vi "F Dwf Analog Impedance Comp Set.vi"(6 "ohmShortReactance":dbl, 7 "ohmShortResistance":dbl, 8 "error in (no error)":errorcluster, 9 "ohmOpenReactance":dbl, 10 "ohmOpenResistance":dbl, 11 "hdwf":i32) -> (0 "error out":errorcluster, 3 "function return":i32)   [LabVIEW 2021, in "Olasdwf.lvlib"]
doc: "DWFAPI int FDwfAnalogImpedanceCompSet(HDWF hdwf, double ohmOpenResistance, double ohmOpenReactance, double ohmShortResistance, double ohmShortReactance);"
uses:
  Olasdwf.lvlib
  Windows/System32/dwf.dll
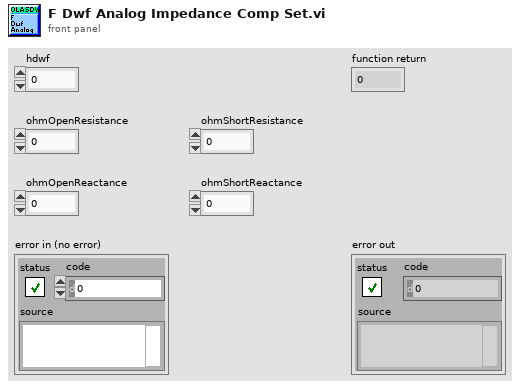
[diagram p1: front panel]
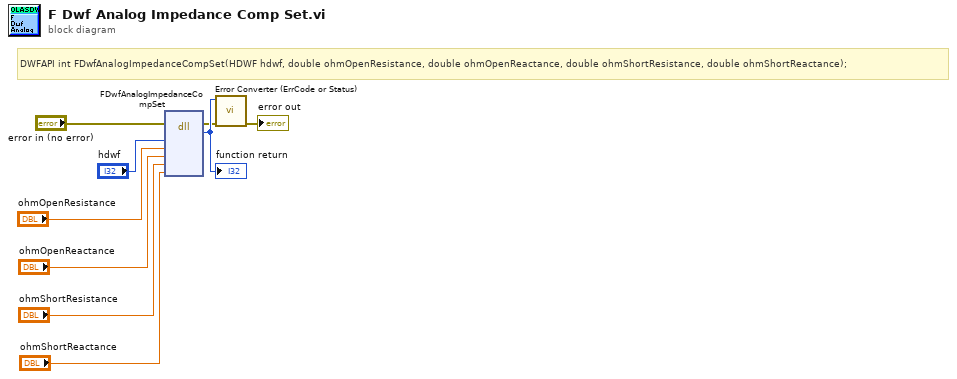
[diagram p0: block diagram]
diagram:
  # "DWFAPI int FDwfAnalogImpedanceCompSet(HDWF hdwf, double ohmOpenResistance, double ohmOpenReactance, double ohmShortResistance, double ohmShortReactance);"
  n1 = dll-call lib="/Windows/System32/dwf.*" fn="FDwfAnalogImpedanceCompSet"(error in="error in (no error)", "hdwf"="hdwf", "ohmOpenResistance"="ohmOpenResistance", "ohmOpenReactance"="ohmOpenReactance", "ohmShortResistance"="ohmShortResistance", "ohmShortReactance"="ohmShortReactance") -> (error out=w2:errorcluster, w9:i32)  [unwired: 7 in, 1 out]
  "function return" <- w9
  n2 = call "Error Converter (ErrCode or Status).vi"("error in (no error)"=w2, "error code"=w9) -> ("error out"=→"error out":errorcluster)  [unwired: 9 in]
